vi "calc calib values from fitting (SubVI).vi"(4 "mag correct":dbl=1.0, 5 "# of slices":i32, 6 "man x correct":dbl[](array[numeric]) format="%_4g", 7 "# of pages":i32, 8 "volume index":i32, 9 "Cluster":T1, 10 "img scan voltage":dbl[][](array[numeric]), 11 "img scan tangent":dbl[][](array[numeric])) -> (3 "Array":dbl[][][](array[numeric]))   [LabVIEW 2024]
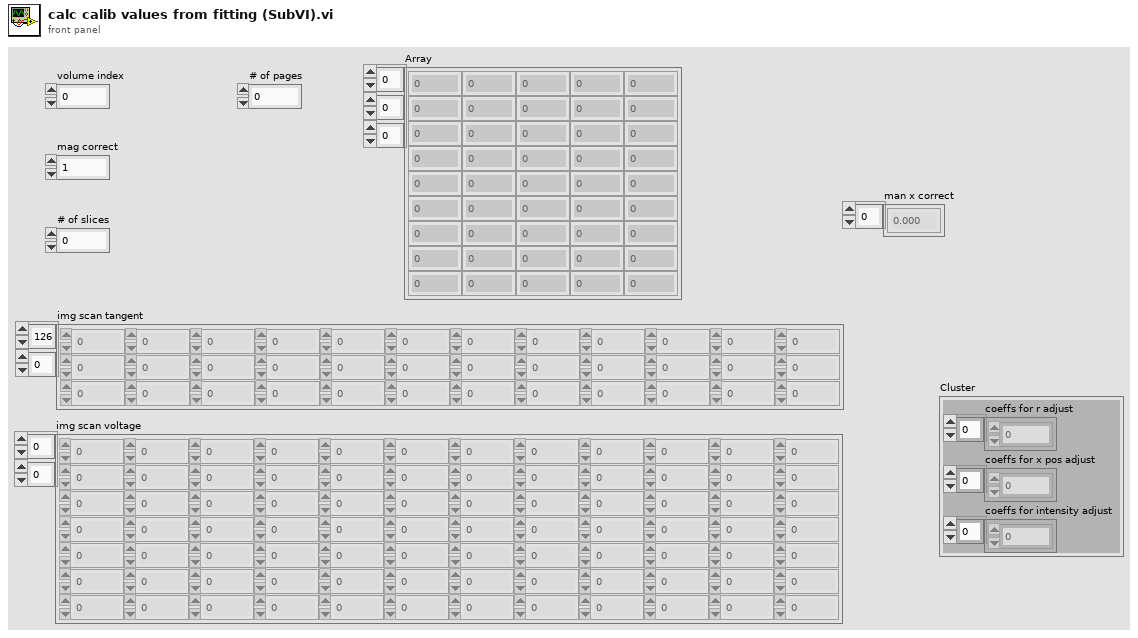
[diagram p1: front panel]
types:
  T1 = cluster{"coeffs for r adjust":dbl[], "coeffs for x pos adjust":dbl[], "coeffs for intensity adjust":dbl[]}
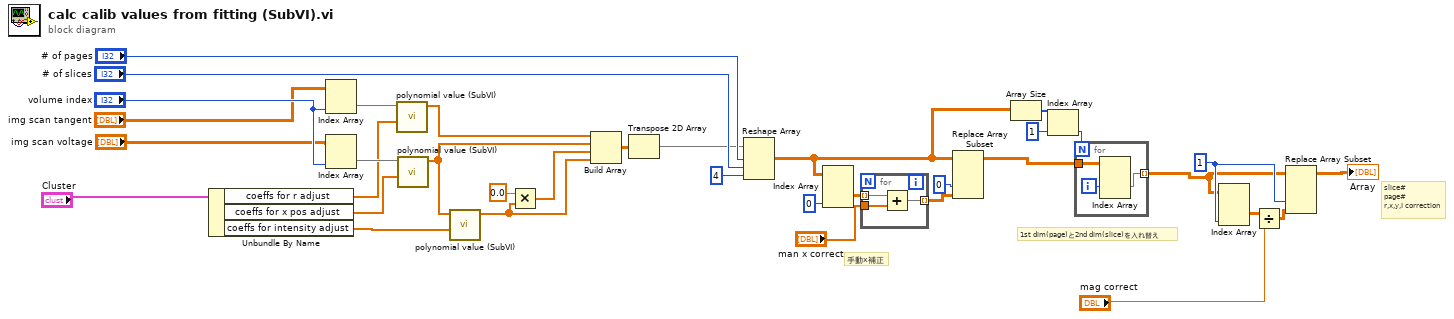
[diagram p0: block diagram]
diagram:
  w5 = 1 ("disabled index (col)")
  # "slice#\npage#\nr,x,y,I correction"
  # "手動x補正"
  # "1st dim(page)と2nd dim(slice)を入れ替え"
  n1 = Unbundle By Name("Cluster") -> ("coeffs for r adjust"=w23:dbl[], "coeffs for x pos adjust"=w25:dbl[], "coeffs for intensity adjust"=w26:dbl[])
  n2 = Index Array(array="img scan tangent", index (col)="volume index") -> (element=w22:dbl[])  [unwired: 1 in]
  n3 = Index Array(array="img scan voltage", index (col)="volume index") -> (element=w24:dbl[])  [unwired: 1 in]
  n4 = call "polynomial value (SubVI).vi"("coeffs"=w23, "x"=w22) -> ("y"=w31:dbl[])  [unwired: 9 in]
  n5 = call "polynomial value (SubVI).vi"("coeffs"=w25, "x"=w24) -> ("y"=w30:dbl[])  [unwired: 9 in]
  n6 = call "polynomial value (SubVI).vi"("coeffs"=w26, "x"=w30) -> ("y"=w29:dbl[])  [unwired: 9 in]
  n7 = Multiply(x=0.0, y=w29) -> (x*y=w28:dbl[])
  n8 = Build Array(w31, w30, w28, w29) -> (w32:dbl[][])
  n9 = Transpose 2D Array(2D array=w32) -> (transposed array=w8:dbl[][])
  n10 = Reshape Array(w8, "# of pages", "# of slices", 4 ("dimension size")) -> (w7:dbl[][][])
  n11 = Index Array(array=w7, index (dim 2)=0 ("disabled index (col)")) -> (element=w14:dbl[][])  [unwired: 2 in]
  n12 = for {
    tunnel: [w38] -> w15 mode=indexing
    tunnel: w14 -> [w37] mode=indexing
    tunnel: "man x correct" -> [w36]
    n13 = Add(x=w37, y=w36) -> (x+y=w38:dbl[])
  }
  n14 = Replace Array Subset(array=w7, new element=w15, index (dim 2)=0 ("disabled index (col)")) -> (w12:dbl[][][])  [unwired: 2 in]
  n15 = Array Size(array=w7) -> (size(s)=w11:i32[])
  n16 = Index Array(array=w11, index=1) -> (element=w9:i32)
  n17 = for {
    N: w9 -> [_]
    tunnel: w12 -> [w41]
    tunnel: [w39] -> w3 mode=indexing
    i -> [w40]
    n18 = Index Array(array=w41, index (dim 1)=w40) -> (element=w39:dbl[][])  [unwired: 2 in]
  }
  n19 = Index Array(array=w3, index (dim 2)=w5) -> (element=w6:dbl[][])  [unwired: 2 in]
  n20 = Divide(x=w6, y="mag correct") -> (x/y=w4:dbl[][])
  n21 = Replace Array Subset(array=w3, new element=w4, index (dim 2)=w5) -> (→"Array":dbl[][][])  [unwired: 2 in]
